vi "Send Finished.vi"(8 "error in (no error)":errorcluster, 9 "Final Error":errorcluster, 10 "Final Actor State":refnum<class "Actor.lvclass">, 11 "Actor-Interface in":refnum<data-value>) -> (0 "error out":errorcluster, 3 "Actor-Interface out":refnum<data-value>)   [LabVIEW 2018, in "Actor.lvlib" / "Actor-Interface.lvclass"]
uses:
  Actor-Interface.lvclass
  Actor.lvclass
  Finished.ctl
  Actor-Interface.lvclass/Actor-Interface.ctl
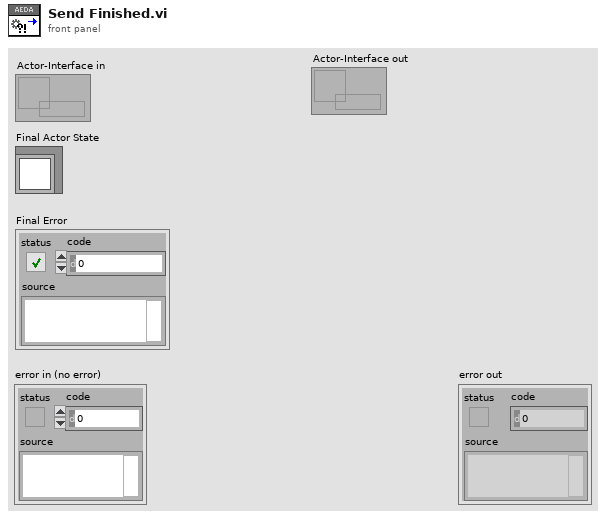
[diagram p1: front panel]
types:
  T1 = typedef "Actor.lvlib/Actor-Interface.lvclass/Finished.ctl" = cluster{"Actor":refnum<class "Actor.lvclass">, "Final Error":errorcluster}
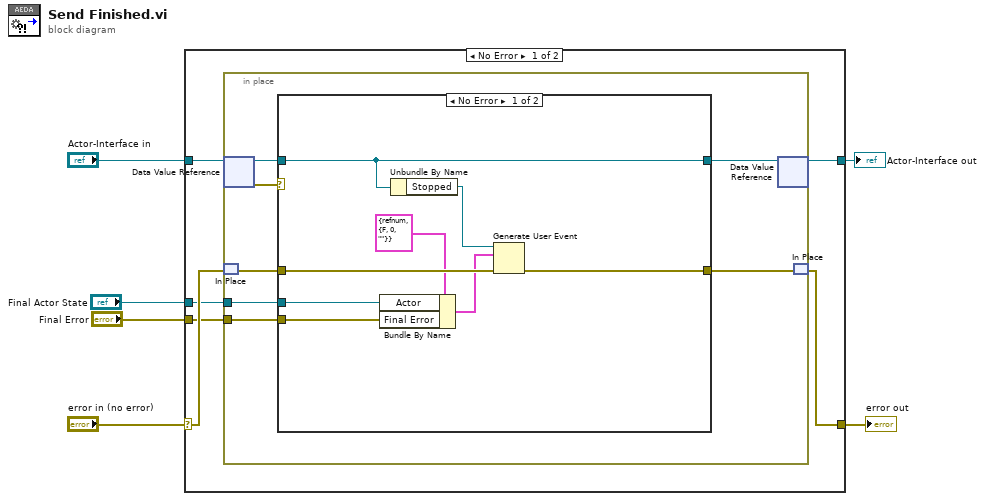
[diagram p0: block diagram]
diagram:
  n1 = case shown="No Error" "error in (no error)" {
    selector: "error in (no error)" -> [w11 w31]
    tunnel: [w7 w31] -> w5
    tunnel: [w8 w30] -> w1
    tunnel: "Actor-Interface in" -> [w12 w30]
    tunnel: "Final Actor State" -> [w10 _]
    tunnel: "Final Error" -> [w9 _]
    frame No Error {
      n2 = in-place {
        in-place-border: w10 -> [w15]
        in-place-border: w9 -> [w14]
        n3 = in-place-dvr #1(w12) -> (w18:refnum<class "Actor-Interface.lvclass">, w19:errorcluster)
        n4 = in-place-match #2(w11) -> (w16:errorcluster)
        n5 = case shown="No Error" w19 {
          tunnel: w18 -> [w27 w29]
          tunnel: [w27 w29] -> w17
          tunnel: w16 -> [w25 w28]
          tunnel: w15 -> [w22 _]
          tunnel: w14 -> [w21 _]
          tunnel: [w20 w28] -> w13
          frame No Error {
            n6 = Bundle By Name(cluster=T1 {"Actor"=refnum, "Final Error"={"status"=FALSE, "code"=0, "source"=""}} ("event data"), "Actor"=w22, "Final Error"=w21) -> (w23:T1)
            n7 = Unbundle By Name(w27) -> ("Stopped"=w26:refnum<user-event>)
            n8 = Generate User Event(user event=w26, event data cluster=w23, error in=w25) -> (error out=w20:errorcluster)  [unwired: 1 in, 1 out]
          }
          frame Error {
          }
        }
        n9 = in-place-dvr #1(w17) -> (w8:refnum<data-value>)  [unwired: 1 out]
        n10 = in-place-match #2(w13) -> (w7:errorcluster)
      }
    }
    frame Error {
    }
  }
  "error out" <- w5
  "Actor-Interface out" <- w1
